vi "Thermal Shock.vi"() -> ()   [LabVIEW 2017]
uses:
  StateDef.ctl
  Thermal Shock.lvlib
panel:
  in  "Tab Control":enum32{"Main Program", "Graph", "Debug"}(tab)
  in  "ProgramTemp":bool
  in  "StopCycling":bool
  in  "StartCycling":bool
  in  "StartChamber":enum32{"Hot", "Cold"}(radio) caption="Starting Chamber"
  in  "Number of Cycles":u32
  in  "Basket Control":enum32{"Basket Up", "Basket Down"}(radio)=enum."Basket Down"
  in  "Stop Recording":bool
  in  "StartRecording":bool
  in  "Recording Interval":T1
  in  "Recording Duration":T2
  in  "Close Program":bool
  out "experiorLogo":picture
  out "Test Information":T3
  in  "HotSetPoint":i32 caption="Hot Chamber Temp (°C)"
  in  "ColdSetPoint":i32 caption="Cold Chamber Temp (°C)"
  in  "ChamberDwells":T4 {"sec_HotDwell" max=60}
  out "TempChart":cluster{"Value":dbl, "Value":i32}[](graph)
  out "Cold Chamber Set Command":string
  out "Hot Chamber Set Command":string
  out "Chamber Dwell Params":u32[](array[numeric])
  out "DataFilePath":path
  in  "Current Temperature":i32[](array[numeric])
  in  "Time (hours)":dbl[](array[numeric])
  out "ElapsedTimeHours":dbl
  out "CurrentColdTemp":i32
  out "CurrentHotTemp":i32
  out "UpdateGraph":bool
  out "FileCreated":bool
  out "CurrentCycle":u32
  out "CycleStartTime":u32
  out "StartTimeDuration":u32
  out "NumberCycles":u32
  out "ColdDwell":u32
  out "HotDwell":u32
  out "Cycling":bool
  out "Close Data Loop":bool
  out "Basket State":u32
  out "Temperature Readings":T5
  out "Data Recording":bool
  out "Recording Interval and Duration":u32[](array[numeric]) caption="MeasParams"
  out "Termination Message":string
  out "Simulated Data":bool
  in  "Queue Cluster":T7
  out "error out":errorcluster
  out "refnum out":refnum<file>
  out "StartTime":u32
  # "File Recording Setup"
  # "Temperature Control"
  # "Cycle Control"
  # "Basket Control"
  # "Data File Information"
  # "Hot Chamber Dwell"
  # "Cold Chamber Dwell"
  # "Temperature Graph"
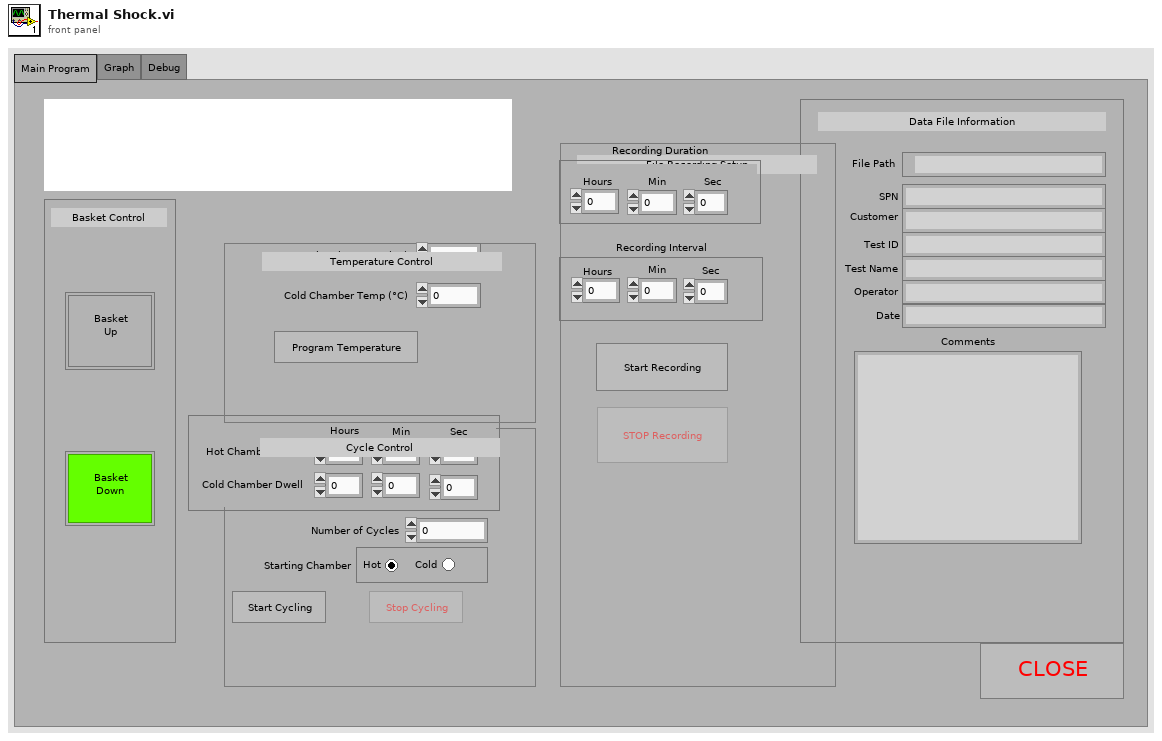
[diagram p1: front panel]
types:
  T1 = cluster{"hours_Interval":i16, "min_Duration":i16, "sec_Duration":i16}
  T2 = cluster{"hours_Duration":u16, "min_Duration":u16, "sec_Duration":i16}
  T3 = cluster{"Test ID":string, "Test Name":string, "Customer":string, "SPN":string, "Operator":string, "Date":string, "File Path":path, "Comments":string}
  T4 = cluster{"hours_HotDwell":u32, "min_HotDwell":u32, "sec_HotDwell":u32, "sec_ColdDwell":u32, "min_ColdDwell":u32, "hours_ColdDwell":u32}
  T5 = cluster{"HotChamber":string, "ColdChamber":string, "Time":string, "Date":string}
  T6 = typedef "StateDef.ctl" = enum16{"Timeout", "AppendFileHeaders", "StopRecording", "TestInformation", "Terminate", "Initialize", "StartRecording", "ReadInstruments", "ReadTemperature", "WriteData", "StartCycling", "StopCycling", "ProgramTemperatures", "CycleBasket"}
  T7 = cluster{"Enum":T6, "Error Note":string, "Message Data":variant}
  T8 = enum8{"Enabled", "Disabled", "Disabled and Grayed Out"}
  T9 = enum16{"open", "replace", "create", "open or create", "replace or create", "replace or create with confirmation"}
  T10 = cluster{string, string, string, string, string, string, path, string}
  T11 = cluster{"Enum":T6, string, "Message Data":variant}
  T12 = cluster{"Test ID":string, "Test Name":string, "Customer":string, "SPN":string, "Operator Name":string, "Date":string, "File Path":path, "Comments":string}
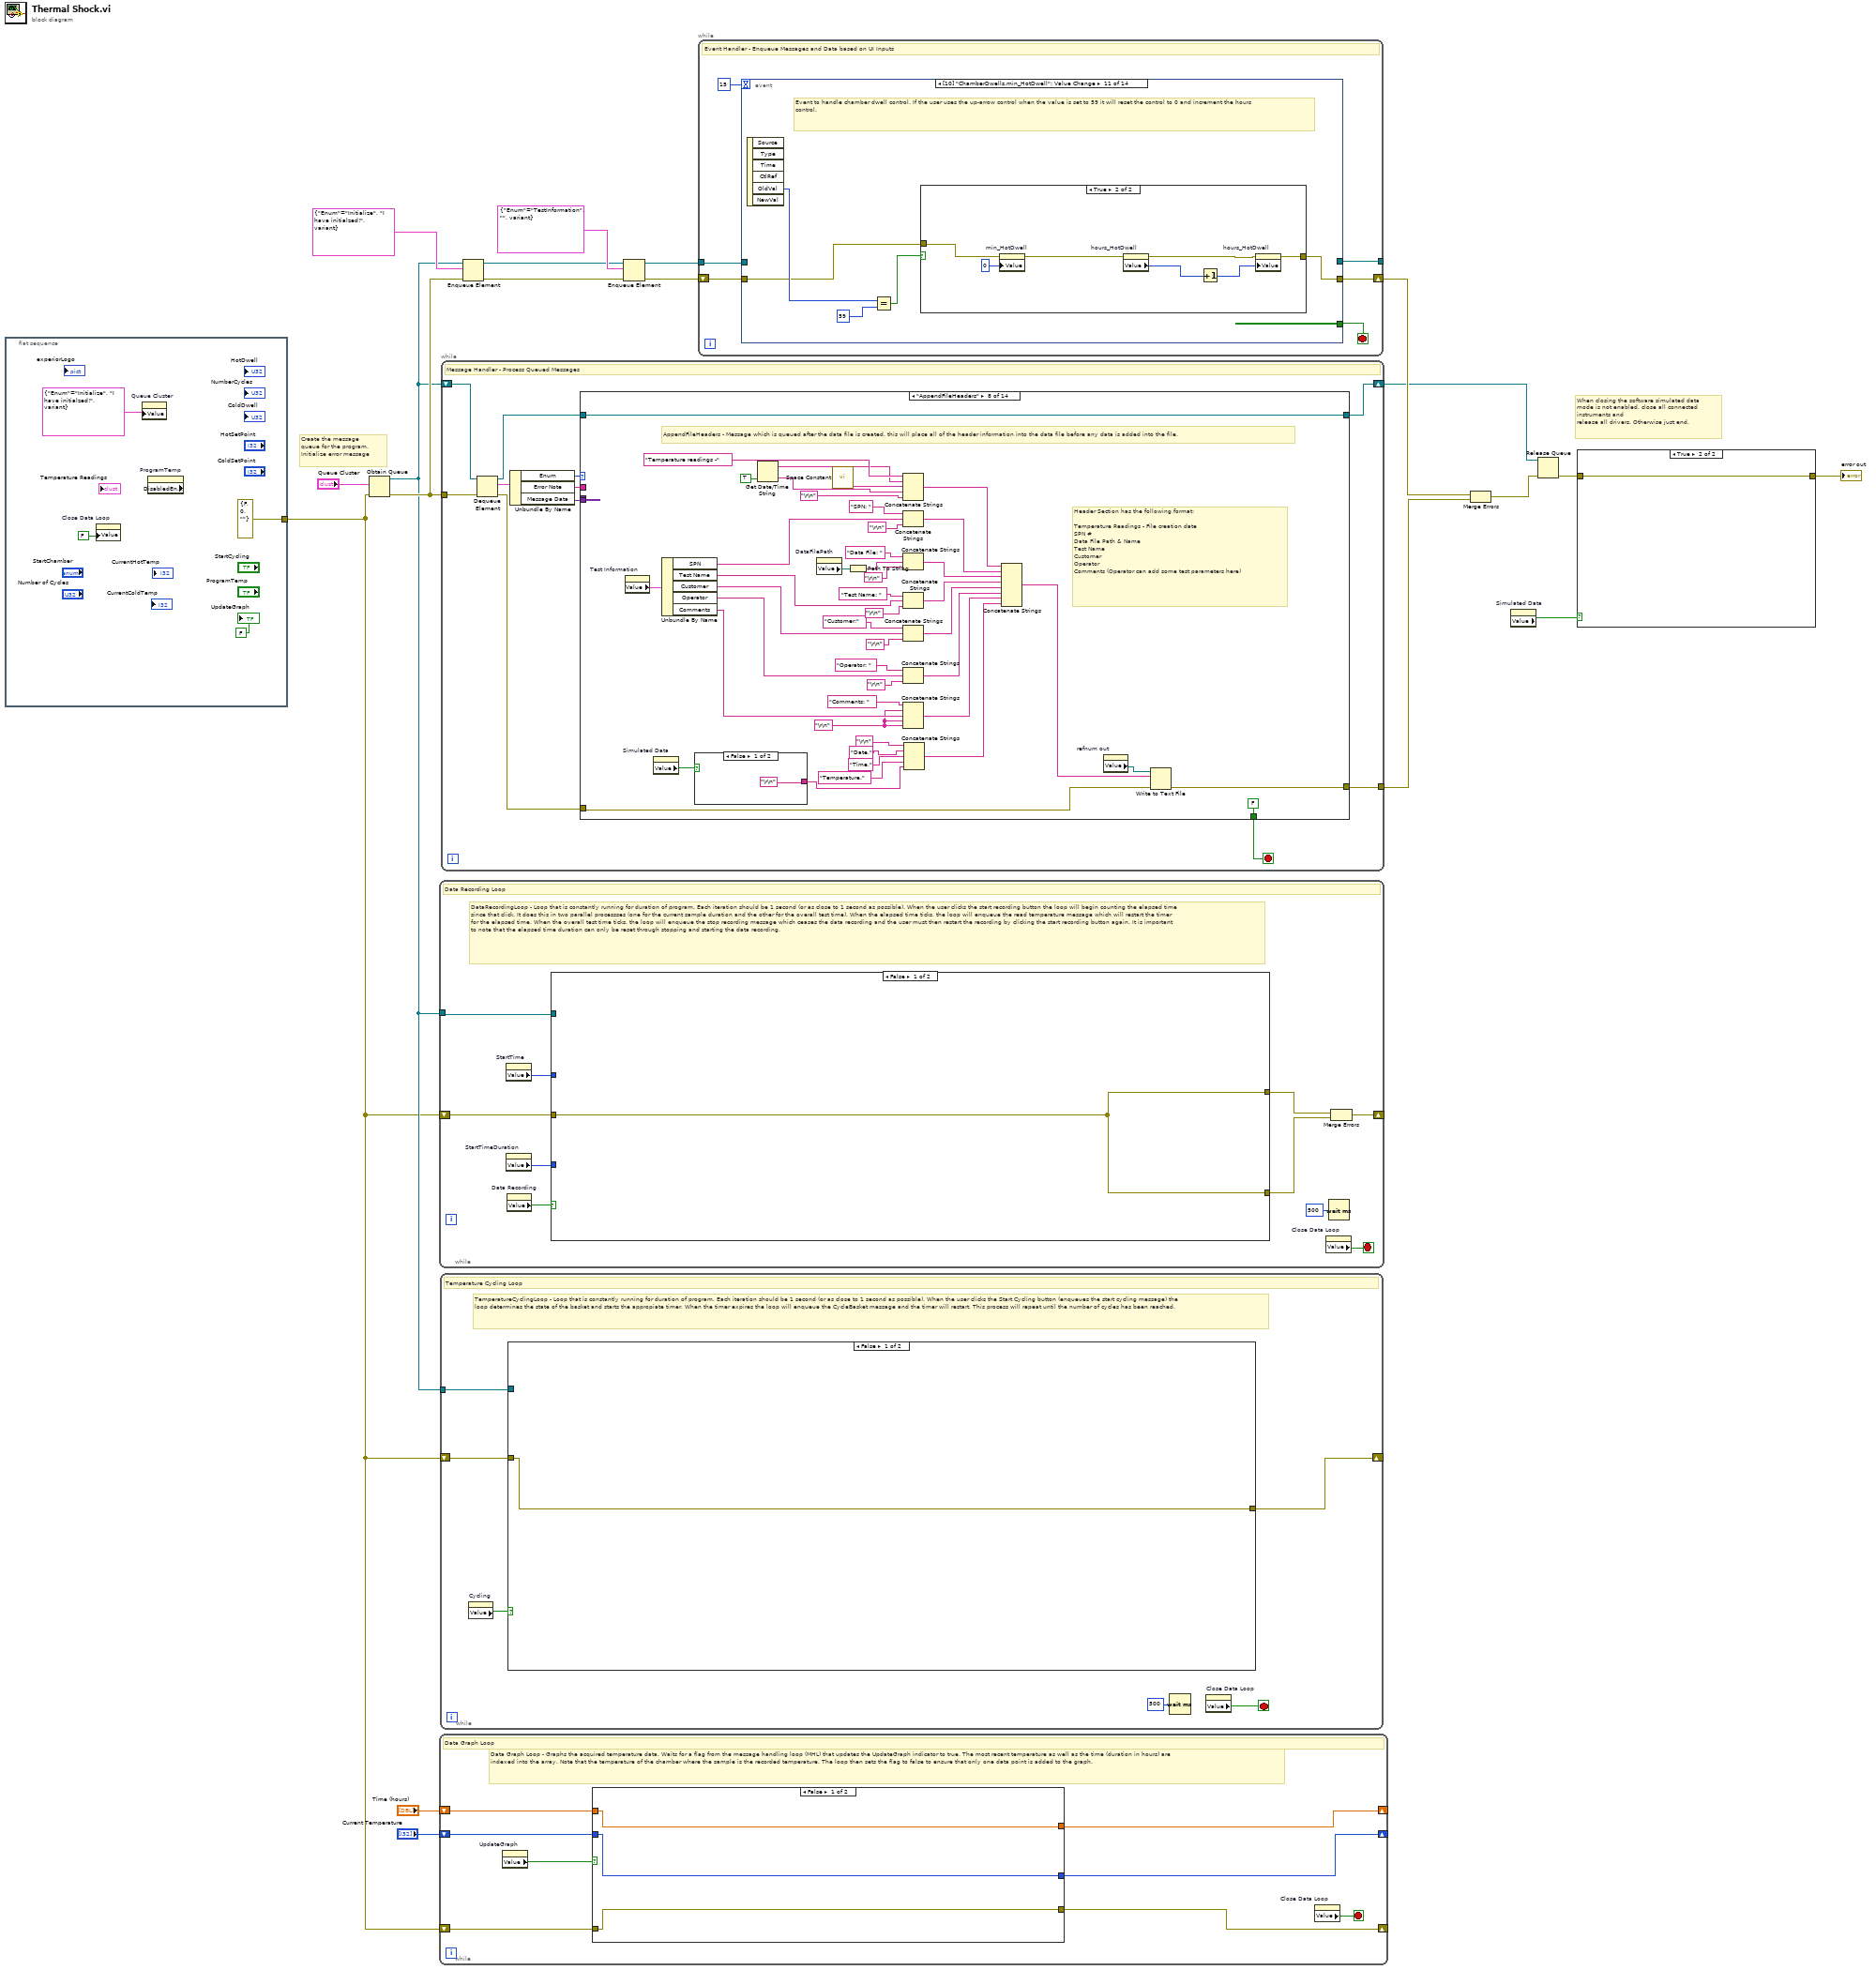
[diagram p0: block diagram]
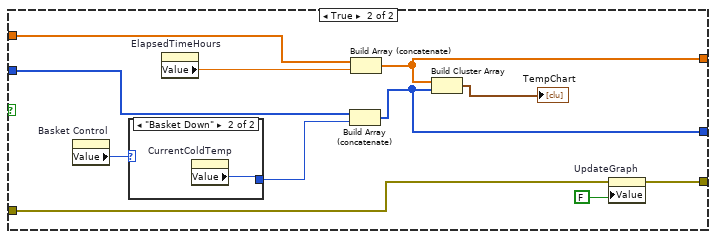
[diagram p2: hidden frame]
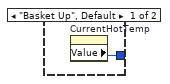
[diagram p3: hidden frame]
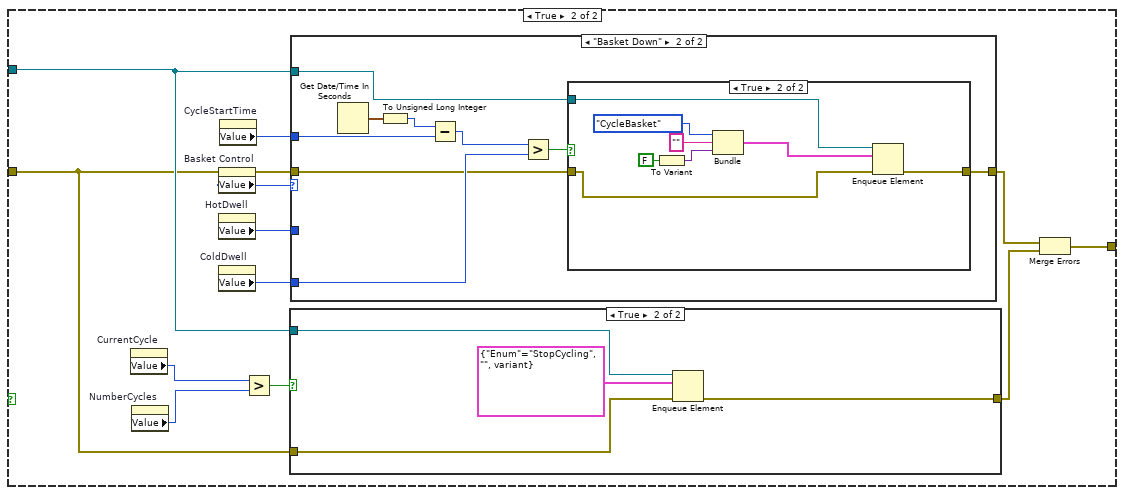
[diagram p4: hidden frame]
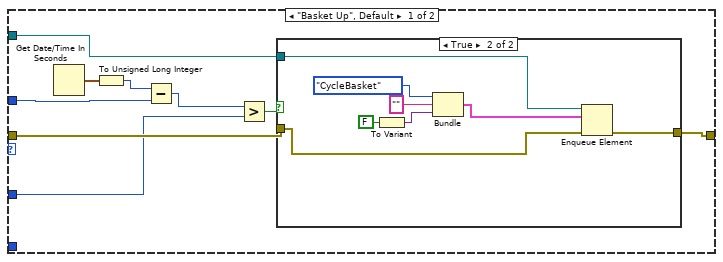
[diagram p6: hidden frame]
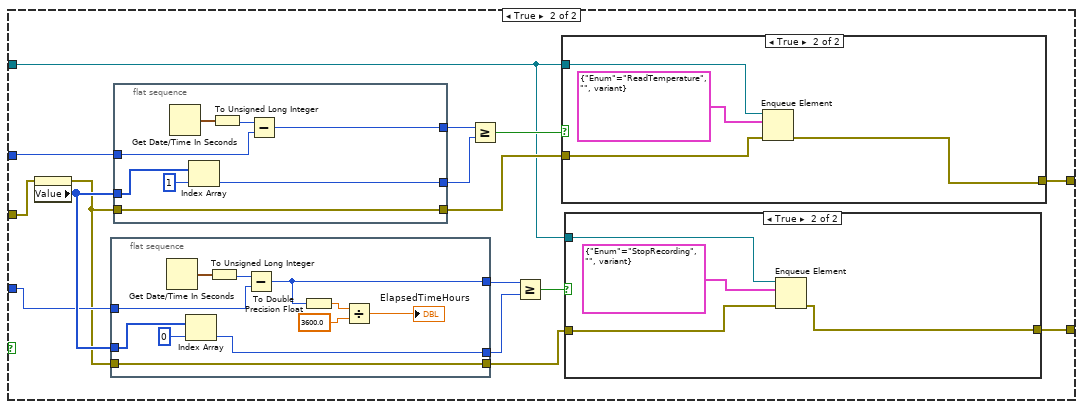
[diagram p9: hidden frame]
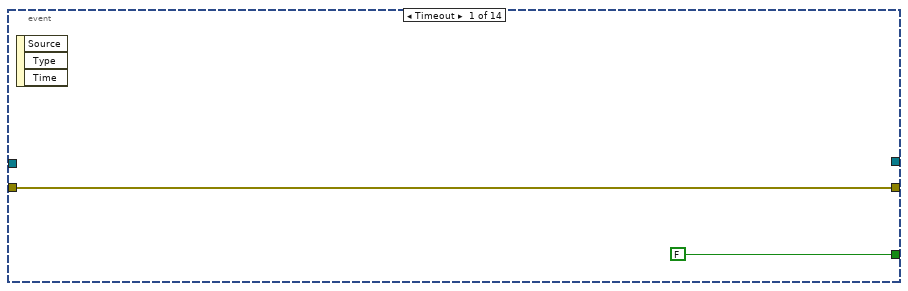
[diagram p13: hidden frame]
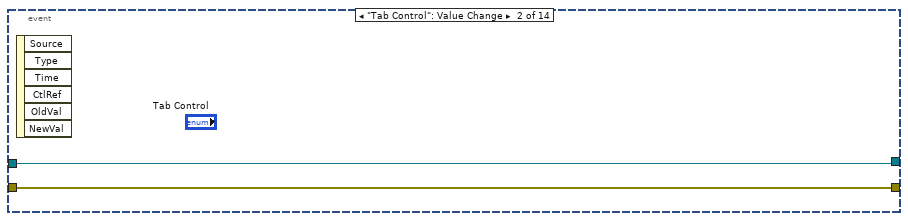
[diagram p14: hidden frame]
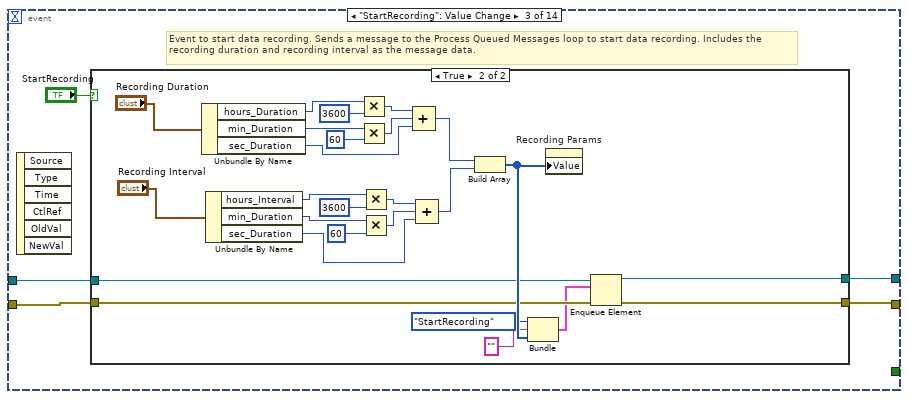
[diagram p15: hidden frame]
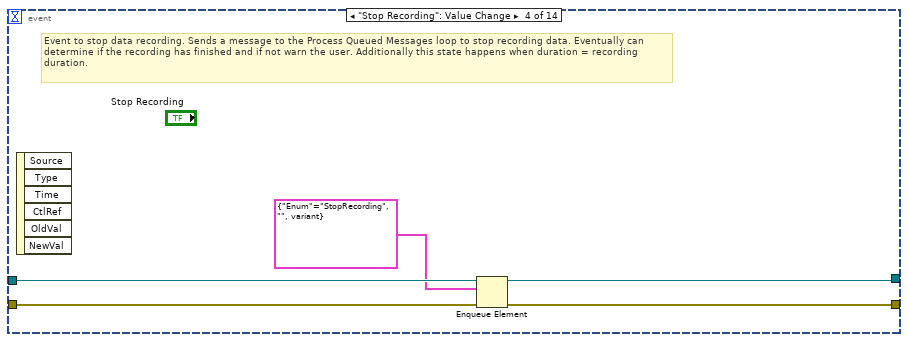
[diagram p17: hidden frame]
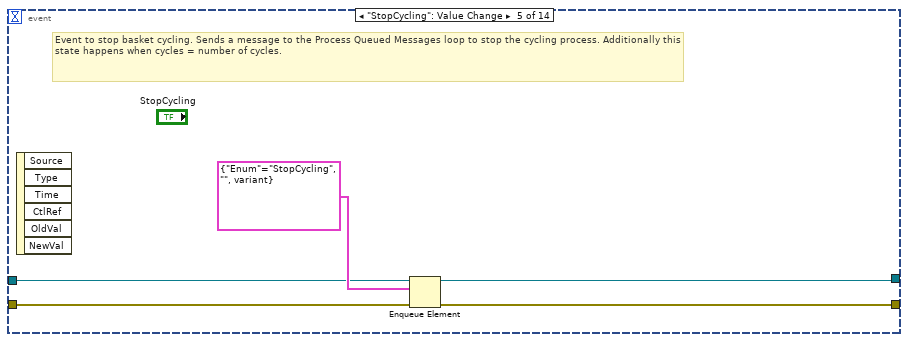
[diagram p18: hidden frame]
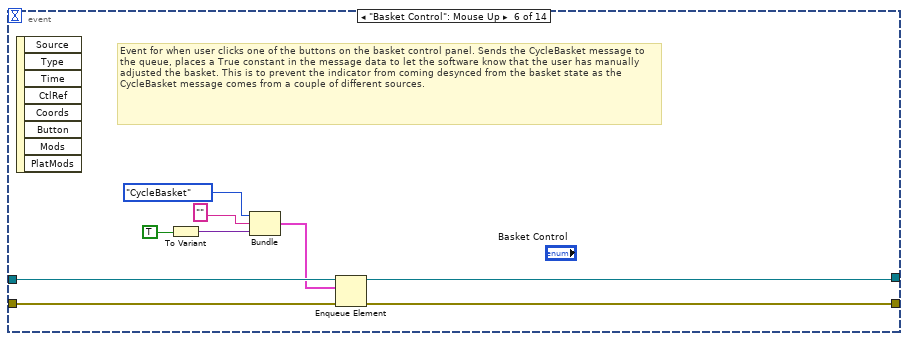
[diagram p19: hidden frame]
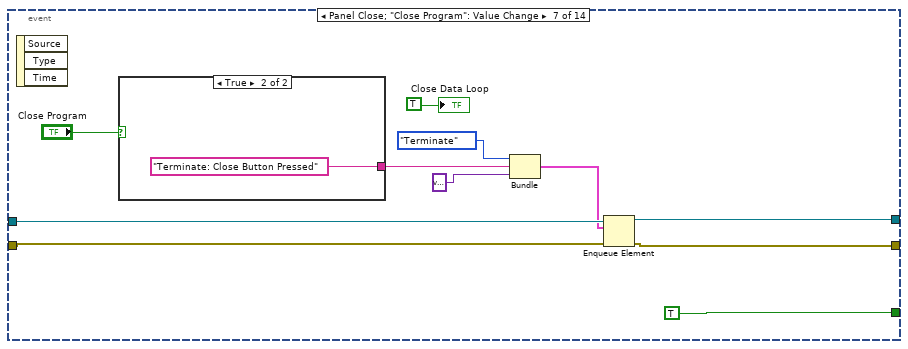
[diagram p20: hidden frame]
diagram:
  # "When closing the software simulated data mode is not enabled, close all connected instruments and \nrelease all drivers. Otherwise just end."
  # "Create the message queue for the program. Initialize error message"
  n1 = flat-sequence {
    tunnel: [errorcluster {"status"=FALSE, "code"=0, "source"=""} ("error constant")] -> w3
    frame #0 {
      n2 = property on="Close Data Loop" class="Bool (strict)"("Value"=FALSE) -> ()  [unwired: 2 in, 2 out]
      n3 = property on="Queue Cluster" class="Clust (strict)"("Value"=cluster{"Enum":T6, string, variant} {"Enum"=enum."Initialize", "I have initialzed!", variant}) -> ()  [unwired: 2 in, 2 out]
      n4 = property on="ProgramTemp" class="Bool" props=["DisabledEnum"]() -> ()  [unwired: 2 in, 3 out]
      "UpdateGraph" <- FALSE ("UpdateGraph")
    }
  }
  n5 = Obtain Queue(element data type="Queue Cluster", error in (no error)=w3) -> (queue out=w4:refnum<queue>, error out=w6:errorcluster)  [unwired: 3 in, 1 out]
  n6 = while {
    shift-right: [w24] -> _
    shift-left: w3 -> [w32]
    tunnel: w4 -> [w31]
    stop <- w28 stop-if-true
    # "DataRecordingLoop - Loop that is constantly running for duration of program. Each iteration should be 1 second (or as close to 1 second as possible). When the user clicks the start recording button the loop will begin counting the elapsed time since that click. It does this in two parallel processses (one for the current sample duration and the other for the overall test time). When the elapsed time ticks, the loop will enqueue the read temperature message which will restart the timer for the elapsed time. When the overall test time ticks, the loop will enqueue the stop recording message which ceases the data recording and the user must then restart the recording by clicking the start recording button again. It is important to note that the elapsed time duration can only be reset through stopping and starting the data recording."
    # "Data Recording Loop"
    n7 = property on="StartTime" class="DigNum (strict)"() -> ("Value"=w29:u32)  [unwired: 2 in, 2 out]
    n8 = property on="StartTimeDuration" class="DigNum (strict)"() -> ("Value"=w27:u32)  [unwired: 2 in, 2 out]
    n9 = property on="Data Recording" class="Bool (strict)"() -> ("Value"=w33:bool)  [unwired: 2 in, 2 out]
    n10 = case shown="False" w33 {
      tunnel: w29 -> [_ w48]
      tunnel: w32 -> [w34 w50]
      tunnel: w31 -> [_ w38]
      tunnel: [w34 w47] -> w26
      tunnel: w27 -> [_ w43]
      tunnel: [w34 w36] -> w25
      frame False {
      }
      frame True {
        n11 = property on="Recording Interval and Duration" class="Arr (strict)"(error in=w50) -> (error out=w42:errorcluster, "Value"=w44:u32[])  [unwired: 1 in, 1 out]
        n12 = flat-sequence {
          tunnel: [w59] -> w41
          tunnel: w43 -> [w64]
          tunnel: w42 -> [w60]
          tunnel: w44 -> [w62]
          tunnel: [w61] -> w40
          tunnel: [w60] -> w37
          frame #0 {
            n13 = Get Date/Time In Seconds() -> (seconds since 1Jan1904=w66:timestamp)
            n14 = Index Array(array=w62, index=0) -> (element=w61:u32)
            n15 = To Unsigned Long Integer(number=w66) -> (unsigned 32bit integer=w65:u32)
            n16 = Subtract(x=w65, y=w64) -> (x-y=w59:u32)
            n17 = To Double Precision Float(number=w59) -> (double precision float=w58:dbl)
            n18 = Divide(x=w58, y=3600.0) -> (x/y=→"ElapsedTimeHours":dbl)
          }
        }
        n19 = flat-sequence {
          tunnel: [w73] -> w35
          tunnel: w48 -> [w71]
          tunnel: w42 -> [w70]
          tunnel: [w70] -> w46
          tunnel: w44 -> [w68]
          tunnel: [w67] -> w45
          frame #0 {
            n20 = Get Date/Time In Seconds() -> (seconds since 1Jan1904=w74:timestamp)
            n21 = Index Array(array=w68, index=1) -> (element=w67:u32)
            n22 = To Unsigned Long Integer(number=w74) -> (unsigned 32bit integer=w72:u32)
            n23 = Subtract(x=w72, y=w71) -> (x-y=w73:u32)
          }
        }
        n24 = Greater Or Equal?(x=w35, y=w45) -> (x >= y?=w49:bool)
        n25 = Greater Or Equal?(x=w41, y=w40) -> (x >= y?=w39:bool)
        n26 = case shown="True" w49 {
          tunnel: w46 -> [w75 w78]
          tunnel: w38 -> [_ w79]
          tunnel: [w75 w77] -> w47
          frame False {
          }
          frame True {
            n27 = Enqueue Element(queue=w79, element=cluster{"Enum":T6, string, variant} {"Enum"=enum."ReadTemperature", "", variant}, error in (no error)=w78) -> (error out=w77:errorcluster)  [unwired: 1 in, 2 out]
          }
        }
        n28 = case shown="True" w39 {
          tunnel: w38 -> [_ w55]
          tunnel: w37 -> [w51 w53]
          tunnel: [w51 w52] -> w36
          frame False {
          }
          frame True {
            n29 = Enqueue Element(queue=w55, element=cluster{"Enum":T6, string, variant} {"Enum"=enum."StopRecording", "", variant}, error in (no error)=w53) -> (error out=w52:errorcluster)  [unwired: 1 in, 2 out]
          }
        }
      }
    }
    n30 = property on="Close Data Loop" class="Bool (strict)"() -> ("Value"=w28:bool)  [unwired: 2 in, 2 out]
    n31 = Wait (ms)(milliseconds to wait=u32 500) -> ()  [unwired: 1 out]
    n32 = Merge Errors(w26, w25) -> (w24:errorcluster)
  }
  n33 = while {
    shift-right: [w84] -> _
    shift-left: w3 -> [w85]
    shift-right: [w80] -> _
    shift-left: "Current Temperature" -> [w82]
    shift-right: [w81] -> _
    shift-left: "Time (hours)" -> [w83]
    stop <- w87 stop-if-true
    # "Data Graph Loop - Graphs the acquired temperature data. Waits for a flag from the message handling loop (MHL) that updates the UpdateGraph indicator to true. The most recent temperature as well as the time (duration in hours) are indexed into the array. Note that the temperature of the chamber where the sample is the recorded temperature. The loop then sets the flag to false to ensure that only one data point is added to the graph."
    # "Data Graph Loop"
    n34 = property on="UpdateGraph" class="Bool (strict)"() -> ("Value"=w86:bool)  [unwired: 2 in, 2 out]
    n35 = case shown="False" w86 {
      tunnel: w85 -> [w90 w100]
      tunnel: [w90 w99] -> w84
      tunnel: w83 -> [w88 w98]
      tunnel: w82 -> [w89 w96]
      tunnel: [w88 w94] -> w81
      tunnel: [w89 w93] -> w80
      frame False {
      }
      frame True {
        n36 = property on="Basket Control" class="RadioBtnsControl (strict)"() -> ("Value"=w91:enum32{"Basket Up", "Basket Down"})  [unwired: 2 in, 2 out]
        n37 = case shown="\"Basket Down\"" w91 {
          tunnel: [w102 w103] -> w95
          frame "Basket Up", Default {
            n38 = property on="CurrentHotTemp" class="DigNum (strict)"() -> ("Value"=w102:i32)  [unwired: 2 in, 2 out]
          }
          frame "Basket Down" {
            n39 = property on="CurrentColdTemp" class="DigNum (strict)"() -> ("Value"=w103:i32)  [unwired: 2 in, 2 out]
          }
        }
        n40 = property on="ElapsedTimeHours" class="DigNum (strict)"() -> ("Value"=w97:dbl)  [unwired: 2 in, 2 out]
        n41 = Build Array (concatenate)(w96, w95) -> (w93:i32[])
        n42 = Build Array (concatenate)(w98, w97) -> (w94:dbl[])
        n43 = Build Cluster Array(w94, w93) -> (→"TempChart":cluster{"Value":dbl, "Value":i32}[])
        n44 = property on="UpdateGraph" class="Bool (strict)"(error in=w100, "Value"=FALSE) -> (error out=w99:errorcluster)  [unwired: 1 in, 1 out]
      }
    }
    n45 = property on="Close Data Loop" class="Bool (strict)"() -> ("Value"=w87:bool)  [unwired: 2 in, 2 out]
  }
  n46 = while {
    tunnel: w4 -> [w107]
    shift-right: [w104] -> _
    shift-left: w3 -> [w106]
    stop <- w109 stop-if-true
    # "TemperatureCyclingLoop - Loop that is constantly running for duration of program. Each iteration should be 1 second (or as close to 1 second as possible). When the user clicks the Start Cycling button (enqueues the start cycling message) the loop determines the state of the basket and starts the appropiate timer. When the timer expires the loop will enqueue the CycleBasket message and the timer will restart. This process will repeat until the number of cycles has been reached."
    # "Temperature Cycling Loop"
    n47 = property on="Cycling" class="Bool (strict)"() -> ("Value"=w105:bool)  [unwired: 2 in, 2 out]
    n48 = case shown="False" w105 {
      tunnel: w107 -> [_ w115]
      tunnel: w106 -> [w110 w114]
      tunnel: [w110 w111] -> w104
      frame False {
      }
      frame True {
        n49 = property on="CurrentCycle" class="DigNum (strict)"() -> ("Value"=w118:u32)  [unwired: 2 in, 2 out]
        n50 = property on="NumberCycles" class="DigNum (strict)"() -> ("Value"=w117:u32)  [unwired: 2 in, 2 out]
        n51 = property on="Basket Control" class="RadioBtnsControl (strict)"(error in=w114) -> (error out=w119:errorcluster, "Value"=w123:enum32{"Basket Up", "Basket Down"})  [unwired: 1 in, 1 out]
        n52 = property on="HotDwell" class="DigNum (strict)"() -> ("Value"=w121:u32)  [unwired: 2 in, 2 out]
        n53 = property on="ColdDwell" class="DigNum (strict)"() -> ("Value"=w120:u32)  [unwired: 2 in, 2 out]
        n54 = property on="CycleStartTime" class="DigNum (strict)"() -> ("Value"=w122:u32)  [unwired: 2 in, 2 out]
        n55 = Greater?(x=w118, y=w117) -> (0:w116:bool)
        n56 = case shown="True" w116 {
          tunnel: w115 -> [_ w127]
          tunnel: w114 -> [w124 w126]
          tunnel: [w124 w125] -> w112
          frame False {
          }
          frame True {
            n57 = Enqueue Element(queue=w127, element=cluster{"Enum":T6, string, variant} {"Enum"=enum."StopCycling", "", variant}, error in (no error)=w126) -> (error out=w125:errorcluster)  [unwired: 1 in, 2 out]
          }
        }
        n58 = case shown="\"Basket Down\"" w123 {
          tunnel: w122 -> [w129 w153]
          tunnel: w121 -> [w131 _]
          tunnel: w120 -> [_ w151]
          tunnel: w115 -> [w133 w149]
          tunnel: w119 -> [w132 w148]
          tunnel: [w130 w147] -> w113
          frame "Basket Up", Default {
            n59 = Get Date/Time In Seconds() -> (seconds since 1Jan1904=w137:timestamp)
            n60 = To Unsigned Long Integer(number=w137) -> (unsigned 32bit integer=w136:u32)
            n61 = Subtract(x=w136, y=w129) -> (x-y=w135:u32)
            n62 = Greater?(x=w135, y=w131) -> (0:w134:bool)
            n63 = case shown="True" w134 {
              tunnel: w133 -> [_ w145]
              tunnel: w132 -> [w138 w146]
              tunnel: [w138 w144] -> w130
              frame False {
              }
              frame True {
                n64 = To Variant(anything=FALSE) -> (Variant=w141:variant)
                n65 = Bundle("Enum"=StateDef."CycleBasket", "", "Variant"=w141) -> (w139:cluster{"Enum":T6, string, "Variant":variant})  [unwired: 1 in]
                n66 = Enqueue Element(queue=w145, element=w139, error in (no error)=w146) -> (error out=w144:errorcluster)  [unwired: 1 in, 2 out]
              }
            }
          }
          frame "Basket Down" {
            n67 = Get Date/Time In Seconds() -> (seconds since 1Jan1904=w155:timestamp)
            n68 = To Unsigned Long Integer(number=w155) -> (unsigned 32bit integer=w154:u32)
            n69 = Subtract(x=w154, y=w153) -> (x-y=w152:u32)
            n70 = Greater?(x=w152, y=w151) -> (0:w150:bool)
            n71 = case shown="True" w150 {
              tunnel: w149 -> [_ w163]
              tunnel: w148 -> [w156 w164]
              tunnel: [w156 w162] -> w147
              frame False {
              }
              frame True {
                n72 = To Variant(anything=FALSE) -> (Variant=w158:variant)
                n73 = Bundle("Enum"=StateDef."CycleBasket", "", "Variant"=w158) -> (w157:cluster{"Enum":T6, string, "Variant":variant})  [unwired: 1 in]
                n74 = Enqueue Element(queue=w163, element=w157, error in (no error)=w164) -> (error out=w162:errorcluster)  [unwired: 1 in, 2 out]
              }
            }
          }
        }
        n75 = Merge Errors(w113, w112) -> (w111:errorcluster)
      }
    }
    n76 = Wait (ms)(milliseconds to wait=u32 500) -> ()  [unwired: 1 out]
    n77 = property on="Close Data Loop" class="Bool (strict)"() -> ("Value"=w109:bool)  [unwired: 2 in, 2 out]
  }
  n78 = while {
    shift-right: [w166] -> w13
    shift-left: w4 -> [w175]
    tunnel: w6 -> [w170]
    tunnel: [w168] -> w14
    stop <- w171 stop-if-true
    # "Message Handler - Process Queued Messages"
    n79 = Dequeue Element(queue=w175, error in (no error)=w170) -> (queue out=w167:refnum<queue>, element=w174:T7, error out=w169:errorcluster)  [unwired: 1 in, 1 out]
    n80 = Unbundle By Name(w174) -> ("Enum"=w173:T6, "Error Note"=w172:string, "Message Data"=w165:variant)
    n81 = case shown="\"AppendFileHeaders\"" w173 {
      tunnel: w172 -> [_ w184 _ _ _ _ _ _ _ _ _ _ _ _]
      tunnel: w165 -> [_ _ _ w226 w257 w327 _ _ w462 w485 _ _ _ _]
      tunnel: [FALSE TRUE FALSE FALSE FALSE FALSE FALSE FALSE FALSE FALSE FALSE FALSE FALSE FALSE] -> w171
      tunnel: w169 -> [w177 w182 w209 w225 w263 w325 w360 w407 w464 w479 w524 w531 w551 w558]
      tunnel: [w177 w179 w209 w231 w256 w301 w340 w439 w453 w476 w524 w525 w549 w555] -> w168
      tunnel: w167 -> [w176 w183 w210 w232 w259 w304 w357 w440 w459 w488 w522 w533 w546 w554]
      tunnel: [w176 w183 w210 w232 w255 w304 w339 w440 w459 w488 w522 w533 w546 w554] -> w166
      tunnel: w165 -> [_ _ _ _ _ _ _ _ _ _ _ _ _ _]
      frame "Timeout", Default {
      }
      frame "Terminate" {
        # "Terminate - Message when the program is closed. Closes any open data files and shuts down all running loops (EHL, MHL, DRL, TCL, DGL). Can add other shutdown procedures here later."
        n82 = property on="FileCreated" class="Bool (strict)"(error in=w182) -> (error out=w180:errorcluster, "Value"=w181:bool)  [unwired: 1 in, 1 out]
        n83 = case shown="True" w181 {
          tunnel: w180 -> [w186 w190]
          tunnel: [w186 w188] -> w179
          frame False {
          }
          frame True {
            n84 = property on="refnum out" class="Ref (strict)"() -> ("Value"=w191:refnum<file>)  [unwired: 2 in, 2 out]
            n85 = Close File(refnum=w191, error in=w190) -> (error out=w189:errorcluster)  [unwired: 1 out]
            n86 = property on="FileCreated" class="Bool (strict)"(error in=w189, "Value"=FALSE ("FileCreated")) -> (error out=w188:errorcluster)  [unwired: 1 in, 1 out]
          }
        }
        n87 = property on="Termination Message" class="Str"("Value"=w184) -> ()  [unwired: 2 in, 2 out]
      }
      frame "Initialize" {
        w211 = FALSE ("Simulated Data")
        w215 = ""
        w219 = u32 1
        w207 = u32 0
        # "Initialize Message - This is the first message processed after starting the program. Applies initial conditions for all relevant controls and indicators. Controls are grouped together in the various blocks."
        n88 = property on="Close Program" class="Bool (strict)"("Value"=FALSE) -> ()  [unwired: 2 in, 2 out]
        n89 = Bundle(w219, w207, w207) -> (w218:cluster{u32, u32, u32})  [unwired: 1 in]
        n90 = Bundle(w207, w219, w207) -> (w217:cluster{u32, u32, u32})  [unwired: 1 in]
        n91 = Bundle(u32 1, u32 30, u32 0, u32 0, u32 30, u32 0) -> (w198:cluster{u32, u32, u32, u32, u32, u32})  [unwired: 1 in]
        n92 = property on="Recording Duration" class="Clust (strict)"("Value"=w218) -> ()  [unwired: 2 in, 2 out]
        n93 = property on="Recording Interval" class="Clust (strict)"("Value"=w217) -> ()  [unwired: 2 in, 2 out]
        n94 = property on="Simulated Data" class="Bool (strict)"("Value"=w211) -> ()  [unwired: 2 in, 2 out]
        n95 = property on="ChamberDwells" class="Clust (strict)"("Value"=w198) -> ()  [unwired: 2 in, 2 out]
        n96 = property on="Number of Cycles" class="DigNum (strict)"("Value"=u32 10 ("Number of Cycles")) -> ()  [unwired: 2 in, 2 out]
        n97 = property on="StartChamber" class="RadioBtnsControl (strict)"("Value"=enum32{"Hot", "Cold"}."Hot" ("StartChamber")) -> ()  [unwired: 2 in, 2 out]
        n98 = Bundle(w215, w215, w215, w215, w215, w215, path "", w215) -> (w214:T10)  [unwired: 1 in]
        n99 = property on="StartRecording" class="Bool"("DisabledEnum"=T8."Enabled" ("Disabled")) -> ()  [unwired: 2 in, 2 out]
        n100 = property on="Stop Recording" class="Bool (strict)"("DisabledEnum"=T8."Disabled and Grayed Out" ("Disabled")) -> ()  [unwired: 2 in, 2 out]
        n101 = property on="Test Information" class="Clust (strict)"("Value"=w214) -> ()  [unwired: 2 in, 2 out]
        n102 = property on="StopCycling" class="Bool (strict)"("DisabledEnum"=T8."Disabled and Grayed Out" ("Disabled")) -> ()  [unwired: 2 in, 2 out]
        n103 = property on="StartCycling" class="Bool (strict)"("DisabledEnum"=T8."Enabled" ("Disabled")) -> ()  [unwired: 2 in, 2 out]
        n104 = property on="ColdSetPoint" class="DigNum (strict)"("Value"=10 ("ColdSetPoint")) -> ()  [unwired: 2 in, 2 out]
        n105 = property on="HotSetPoint" class="DigNum (strict)"("Value"=35 ("HotSetPoint")) -> ()  [unwired: 2 in, 2 out]
        "Termination Message" <- ""
        "Data Recording" <- w211
        "Cycling" <- FALSE
        "FileCreated" <- FALSE
      }
      frame "ProgramTemperatures" {
        w227 = 0
        # "ProgramTemperatures - Message which attempts to send the values in the Temperature Control block to the Chromalox controller. The message data is in the format of a 2 Integer cluster with the following structure:\n\nI32[0] = Hot Chamber Temperature\nI32[1] = Cold Chamber Temperature\n\nNote that when the Simulated Data control is enabled this message does nothing (no good way to enable debugging for this method)."
        n106 = property on="Simulated Data" class="Bool (strict)"() -> ("Value"=w233:bool)  [unwired: 2 in, 2 out]
        n107 = Bundle(w227, w227) -> (w228:cluster{i32, i32})  [unwired: 1 in]
        n108 = Variant To Data(error in=w225, type=w228, Variant=w226) -> (data=w229:cluster{i32, i32}, error out=w224:errorcluster)
        n109 = Unbundle(w229) -> (w223:i32, w222:i32)
        n110 = case shown="True" w233 {
          tunnel: w224 -> [w234 w249]
          tunnel: [w237 w249] -> w231
          tunnel: w223 -> [w236 w248]
          tunnel: w222 -> [w235 w247]
          frame False {
            n111 = call "SetHighPoint.vi"("error in (no error)"=w234, "High Temperature"=w236) -> ("error out"=w238:errorcluster)  [unwired: 8 in, 1 out]
            n112 = call "SetLowPoint.vi"("error in (no error)"=w238, "Low Temperature"=w235) -> ("error out"=w237:errorcluster)  [unwired: 8 in, 1 out]
          }
          frame True {
            n113 = call "FormatHexValue.vi"("Value"=w248) -> ("FormattedValue"=w246:string)  [unwired: 10 in]
            n114 = call "FormatHexValue.vi"("Value"=w247) -> ("FormattedValue"=w243:string)  [unwired: 10 in]
            n115 = Concatenate Strings("0108000101", w246) -> (w242:string)
            n116 = Concatenate Strings("0108000201", w243) -> (w241:string)
            n117 = call "ComputeChecksum.vi"("Input Command"=w242) -> ("Command Message"=→"Hot Chamber Set Command":string)  [unwired: 9 in, 1 out]
            n118 = call "ComputeChecksum.vi"("Input Command"=w241) -> ("Command Message"=→"Cold Chamber Set Command":string)  [unwired: 9 in, 1 out]
          }
        }
      }
      frame "StartCycling" {
        # "StartCycling Message - When this message is received the software checks that the basket is in the proper starting chamber, if it is not then it will queue the cycle basket message follwed by the start cycling message so that the basket will be put in the right position. Otherwise this message will start the cycling timer.  This message will also update the status boxes for the two different dwell times and the number of cycles to keep track of where the program is."
        n119 = property on="Basket Control" class="RadioBtnsControl (strict)"() -> ("Value"=w254:enum32{"Basket Up", "Basket Down"})  [unwired: 2 in, 2 out]
        n120 = property on="StartChamber" class="RadioBtnsControl (strict)"() -> ("Value"=w253:enum32{"Hot", "Cold"})  [unwired: 2 in, 2 out]
        n121 = property on="StartCycling" class="Bool (strict)"(error in=w263, "DisabledEnum"=T8."Disabled and Grayed Out" ("Disabled")) -> (error out=w262:errorcluster)  [unwired: 1 in, 1 out]
        n122 = To Unsigned Long Integer(number=w254) -> (unsigned 32bit integer=w252:u32)
        n123 = To Unsigned Long Integer(number=w253) -> (unsigned 32bit integer=w251:u32)
        n124 = Equal?(x=w252, y=w251) -> (x = y?=w250:bool)
        n125 = property on="StopCycling" class="Bool (strict)"(error in=w262, "DisabledEnum"=T8."Enabled" ("Disabled")) -> (error out=w258:errorcluster)  [unwired: 1 in, 1 out]
        n126 = case shown="True" w250 {
          tunnel: w259 -> [w279 w290]
          tunnel: w258 -> [w278 w293]
          tunnel: [w271 w288] -> w256
          tunnel: w257 -> [w275 w291]
          tunnel: [w270 w290] -> w255
          frame False {
            n127 = To Variant(anything=FALSE) -> (Variant=w266:variant)
            n128 = Bundle("Enum"=StateDef."CycleBasket", "", "Variant"=w266) -> (w265:cluster{"Enum":T6, string, "Variant":variant})  [unwired: 1 in]
            n129 = Enqueue Element(queue=w279, element=w265, error in (no error)=w278) -> (queue out=w273:refnum<queue>, error out=w272:errorcluster)  [unwired: 1 in, 1 out]
            n130 = Bundle("Enum"=StateDef."StartCycling", "", "Message Data"=w275) -> (w274:T11)  [unwired: 1 in]
            n131 = Enqueue Element(queue=w273, element=w274, error in (no error)=w272) -> (queue out=w270:refnum<queue>, error out=w271:errorcluster)  [unwired: 1 in, 1 out]
          }
          frame True {
            n132 = property on="Chamber Dwell Params" class="Arr (strict)"() -> ("Value"=w287:u32[])  [unwired: 2 in, 2 out]
            n133 = Variant To Data(error in=w293, type=w287, Variant=w291) -> (data=w286:u32[], error out=w292:errorcluster)
            "Chamber Dwell Params" <- w286
            n134 = Index Array(array=w286, index #1=0 ("index"), index #2=1 ("index"), index #3=2 ("index")) -> (element #1=w282:u32, element #2=w281:u32, element #3=w280:u32)
            n135 = property on="Cycling" class="Bool (strict)"(error in=w292, "Value"=TRUE) -> (error out=w289:errorcluster)  [unwired: 1 in, 1 out]
            n136 = flat-sequence {
              tunnel: w289 -> [w296]
              tunnel: [w296] -> w288
              frame #0 {
                n137 = Get Date/Time In Seconds() -> (seconds since 1Jan1904=w297:timestamp)
                n138 = To Unsigned Long Integer(number=w297) -> (unsigned 32bit integer=→"CycleStartTime":u32)
                "CurrentCycle" <- u32 1
              }
            }
            n139 = property on="ColdDwell" class="DigNum (strict)"("Value"=w281) -> ()  [unwired: 2 in, 2 out]
            n140 = property on="HotDwell" class="DigNum (strict)"("Value"=w282) -> ()  [unwired: 2 in, 2 out]
            n141 = property on="NumberCycles" class="DigNum (strict)"("Value"=w280) -> ()  [unwired: 2 in, 2 out]
          }
        }
      }
      frame "StartRecording" {
        # "Take a timestamp for the start time. The data recording loop iterates every 500ms to check for a tick."
        # "Start Recording message, receives the recording (sampling) interval and recording (sampling) duration, both in seconds. Creates a new data file (csv) every time the start recording button is pressed, the file uses the time stamp to ensure a new file is created for each run. Sets the Data Recording indicator to true which will signal the data recording loop to begin processing."
        n142 = property on="Recording Interval and Duration" class="Arr (strict)"() -> ("Value"=w326:u32[])  [unwired: 2 in, 2 out]
        n143 = Variant To Data(error in=w325, type=w326, Variant=w327) -> (data=→"Recording Interval and Duration":u32[], error out=w313:errorcluster)
        n144 = property on="Test Information" class="Clust (strict)"() -> ("Value"=w322:T3)  [unwired: 2 in, 2 out]
        n145 = property on="StartRecording" class="Bool"(error in=w313, "DisabledEnum"=T8."Disabled and Grayed Out" ("Disabled")) -> (error out=w312:errorcluster)  [unwired: 1 in, 1 out]
        n146 = Unbundle By Name(w322) -> ("File Path"=w321:path, "SPN"=w316:string, "Test ID"=w309:string, "Test Name"=w308:string)
        n147 = call <vilib>:"Space Constant.vi"() -> ("String"=w307:string)
        n148 = Format Date/Time String(time format string (%c)="%Y%m%d%I%M%S") -> (date/time string=w306:string)  [unwired: 2 in]
        n149 = Path To String(path=w321) -> (string=w320:string)
        n150 = property on="Stop Recording" class="Bool (strict)"(error in=w312, "DisabledEnum"=T8."Enabled" ("Disabled")) -> (error out=w311:errorcluster)  [unwired: 1 in, 1 out]
        n151 = Concatenate Strings(w320, "\\", "SPN", w316, w307, w309, w307, w308, w307, w306, ".csv") -> (w318:string)
        n152 = String To Path(string=w318) -> (path=w299:path)
        "DataFilePath" <- w299
        n153 = Open/Create/Replace File(file path (use dialog)=w299, error in=w311, operation (0:open)=T9."create") -> (refnum out=→"refnum out":refnum<file>, error out=w303:errorcluster)  [unwired: 3 in, 1 out]
        n154 = Enqueue Element(queue=w304, element=cluster{"Enum":T6, string, variant} {"Enum"=enum."AppendFileHeaders", "", variant}, error in (no error)=w303) -> (error out=w302:errorcluster)  [unwired: 1 in, 2 out]
        n155 = flat-sequence {
          tunnel: w302 -> [w332]
          tunnel: [w332] -> w301
          frame #0 {
            n156 = Get Date/Time In Seconds() -> (seconds since 1Jan1904=w336:timestamp)
            n157 = Get Date/Time In Seconds() -> (seconds since 1Jan1904=w334:timestamp)
            n158 = To Unsigned Long Integer(number=w336) -> (unsigned 32bit integer=→"StartTime":u32)
            n159 = To Unsigned Long Integer(number=w334) -> (unsigned 32bit integer=→"StartTimeDuration":u32)
            n160 = property on="Data Recording" class="Bool (strict)"("Value"=TRUE) -> ()  [unwired: 2 in, 2 out]
            n161 = property on="FileCreated" class="Bool (strict)"("Value"=TRUE ("FileCreated")) -> ()  [unwired: 2 in, 2 out]
          }
        }
      }
      frame "ReadTemperature" {
        # "NOTE: The read commands for the Chromalox controller only return the offset from the set point temperature. This message reads the set point for each chamber and calculates the current temperature based on the offset. Can optimize by replacing the ReadHighSets with an indicator on the Main VI. \nNOTE2: Currently it seems like the Chromalox can only return/set integer values to/from the chamber. Legacy code was coded in a method that accounts for doubles however I could not find any data to support that. Looking into if this is a limitation of the controller or if there is a method for using doubles. Code is setup for calculating doubles however the values are just casted to 32 bit integers."
        # "Read Temperature Method - currently only called from a tick of the Data Recording Loop. Reads the temperature in the top and bottom chambers and creates a message from the two points. Enqueues the write data message to write the temperature to the data file. Built for expandability for collecting other types of data points."
        n162 = property on="Simulated Data" class="Bool (strict)"(error in=w360) -> (error out=w358:errorcluster, "Value"=w359:bool)  [unwired: 1 in, 1 out]
        n163 = case shown="False" w359 {
          tunnel: w358 -> [w367 w379]
          tunnel: w357 -> [w378 w380]
          tunnel: [w368 w382] -> w344
          tunnel: [w369 w381] -> w345
          tunnel: [w378 w380] -> w342
          tunnel: [w362 w379] -> w341
          frame False {
            n164 = call "ReadLowSetpoint.vi"("error in (no error)"=w367) -> ("error out"=w365:errorcluster, "LowChamberSetPoint"=w375:dbl)  [unwired: 7 in, 2 out]
            n165 = call "ReadHighSetpoint.vi"("error in (no error)"=w367) -> ("error out"=w366:errorcluster, "HighChamberSetPoint"=w377:dbl)  [unwired: 7 in, 2 out]
            n166 = call "ReadLowTemp.vi"("error in (no error)"=w365) -> ("error out"=w363:errorcluster, "CurrentTemp(LowChamber)"=w374:dbl)  [unwired: 7 in, 1 out]
            n167 = call "ReadHighTemp.vi"("error in (no error)"=w366) -> ("error out"=w364:errorcluster, "CurrentTemp(HighChamber)"=w376:dbl)  [unwired: 8 in, 1 out]
            n168 = Subtract(x=w377, y=w376) -> (x-y=w373:dbl)
            n169 = Subtract(x=w375, y=w374) -> (x-y=w372:dbl)
            n170 = To Long Integer(number=w373) -> (32bit integer=w371:i32)
            n171 = To Long Integer(number=w372) -> (32bit integer=w370:i32)
            n172 = Number To Decimal String(number=w371) -> (decimal integer string=w368:string)  [unwired: 1 in]
            n173 = Number To Decimal String(number=w370) -> (decimal integer string=w369:string)  [unwired: 1 in]
            n174 = Merge Errors(w364, w363) -> (w362:errorcluster)
          }
          frame True {
            n175 = Random Number (0-1)() -> (number: 0 to 1=w394:dbl)
            n176 = Random Number (0-1)() -> (number: 0 to 1=w393:dbl)
            n177 = property on="HotSetPoint" class="DigNum (strict)"() -> ("Value"=w388:i32)  [unwired: 2 in, 2 out]
            n178 = property on="ColdSetPoint" class="DigNum (strict)"() -> ("Value"=w386:i32)  [unwired: 2 in, 2 out]
            n179 = Multiply(x=w394, y=2.0) -> (x*y=w390:dbl)
            n180 = Multiply(x=w393, y=2.0) -> (x*y=w389:dbl)
            n181 = To Long Integer(number=w389) -> (32bit integer=w385:i32)
            n182 = To Long Integer(number=w390) -> (32bit integer=w387:i32)
            n183 = Add(x=w388, y=w387) -> (x+y=w384:i32)
            n184 = Add(x=w386, y=w385) -> (x+y=w383:i32)
            n185 = Number To Decimal String(number=w384) -> (decimal integer string=w382:string)  [unwired: 1 in]
            n186 = Number To Decimal String(number=w383) -> (decimal integer string=w381:string)  [unwired: 1 in]
            n187 = property on="CurrentColdTemp" class="DigNum (strict)"("Value"=w383) -> ()  [unwired: 2 in, 2 out]
            n188 = property on="CurrentHotTemp" class="DigNum (strict)"("Value"=w384) -> ()  [unwired: 2 in, 2 out]
          }
        }
        n189 = Get Date/Time String(want seconds? (F)=TRUE) -> (date string=w338:string, time string=w337:string)  [unwired: 2 in]
        n190 = property on="Temperature Readings" class="Clust (strict)"() -> ("Value"=w356:T5)  [unwired: 2 in, 2 out]
        n191 = Bundle By Name(cluster=w356, "HotChamber"=w344, "ColdChamber"=w345, "Date"=w338, "Time"=w337) -> (w355:T5)
        n192 = To Variant(anything=w355) -> (Variant=w354:variant)
        n193 = Bundle("Enum"=StateDef."WriteData", "", "Variant"=w354) -> (w353:cluster{"Enum":T6, string, "Variant":variant})  [unwired: 1 in]
        n194 = Enqueue Element(queue=w342, element=w353, error in (no error)=w341) -> (queue out=w339:refnum<queue>, error out=w350:errorcluster)  [unwired: 1 in, 1 out]
        n195 = property on="UpdateGraph" class="Bool (strict)"(error in=w350, "Value"=TRUE ("UpdateGraph")) -> (error out=w349:errorcluster)  [unwired: 1 in, 1 out]
        n196 = Get Date/Time In Seconds() -> (seconds since 1Jan1904=w351:timestamp)
        n197 = To Unsigned Long Integer(number=w351) -> (unsigned 32bit integer=w352:u32)
        n198 = property on="StartTime" class="DigNum (strict)"(error in=w349, "Value"=w352) -> (error out=w340:errorcluster)  [unwired: 1 in, 1 out]
      }
      frame "AppendFileHeaders" {
        w416 = "\r\n"
        # "Header Section has the following format:\n\nTemperature Readings - File creation date\nSPN #\nData File Path & Name\nTest Name\nCustomer\nOperator\nComments (Operator can add some test parameters here)"
        # "AppendFileHeaders - Message which is queued after the data file is created, this will place all of the header information into the data file before any data is added into the file."
        n199 = property on="Test Information" class="Clust (strict)"() -> ("Value"=w436:T3)  [unwired: 2 in, 2 out]
        n200 = property on="Simulated Data" class="Bool (strict)"() -> ("Value"=w397:bool)  [unwired: 2 in, 2 out]
        n201 = Unbundle By Name(w436) -> ("SPN"=w432:string, "Test Name"=w426:string, "Customer"=w423:string, "Operator"=w421:string, "Comments"=w417:string)
        n202 = case shown="False" w397 {
          tunnel: ["\r\n" w442] -> w395
          frame False {
          }
          frame True {
            n203 = Concatenate Strings(",BasketPosition,", "\r\n") -> (w442:string)
          }
        }
        n204 = Get Date/Time String(want seconds? (F)=TRUE) -> (date string=w404:string, time string=w403:string)  [unwired: 2 in]
        n205 = property on="DataFilePath" class="Path"() -> ("Value"=w437:path)  [unwired: 2 in, 2 out]
        n206 = call <vilib>:"Space Constant.vi"() -> ("String"=w405:string)
        n207 = Path To String(path=w437) -> (string=w429:string)
        n208 = Concatenate Strings("Temperature readings -", w404, w405, w403, "\r\n") -> (w415:string)
        n209 = Concatenate Strings("SPN: ", w432, "\r\n") -> (w414:string)
        n210 = Concatenate Strings("Data File: ", w429, "\r\n") -> (w413:string)
        n211 = Concatenate Strings("Test Name: ", w426, "\r\n") -> (w412:string)
        n212 = Concatenate Strings("Customer:", w423, "\r\n") -> (w411:string)
        n213 = Concatenate Strings("Operator: ", w421, "\r\n") -> (w410:string)
        n214 = Concatenate Strings("Comments: ", w416, w417, w416, w416) -> (w409:string)
        n215 = Concatenate Strings("\r\n", "Date,", "Time,", "Temperature,", w395) -> (w396:string)
        n216 = Concatenate Strings(w415, w414, w413, w412, w411, w410, w409, w396) -> (w408:string)
        n217 = property on="refnum out" class="Ref (strict)"() -> ("Value"=w402:refnum<file>)  [unwired: 2 in, 2 out]
        n218 = Write to Text File(file (use dialog)=w402, text=w408, error in=w407) -> (error out=w439:errorcluster)  [unwired: 1 in, 2 out]
      }
      frame "WriteData" {
        w449 = ","
        # "If the system is in debugging mode (simulated data = true) then the basket state will be written to the data file, otherwise only write the message data."
        # "Message data for the WriteData message is a string cluster with the following structure:\n1. Hot Chamber Temperature\n2. Cold Chamber Temperature\n3. Date\n4. Time\nData is formatted for a csv intput and written to the data file."
        n219 = property on="Simulated Data" class="Bool (strict)"() -> ("Value"=w451:bool)  [unwired: 2 in, 2 out]
        n220 = case shown="True" w451 {
          tunnel: ["\r\n" w473] -> w450
          frame False {
          }
          frame True {
            n221 = property on="Basket Control" class="RadioBtnsControl (strict)"() -> ("Value"=w474:enum32{"Basket Up", "Basket Down"})  [unwired: 2 in, 2 out]
            n222 = Format Into String(w474) -> (resulting string=w471:string)  [unwired: 3 in, 1 out]
            n223 = Concatenate Strings(",", w471, "\r\n") -> (w473:string)
          }
        }
        n224 = Variant To Data(type=cluster{string, string, string, string} {"", "", "", ""}, Variant=w462) -> (data=w461:cluster{string, string, string, string})  [unwired: 1 in, 1 out]
        n225 = Unbundle(w461) -> (w447:string, w446:string, w456:string, w457:string)
        n226 = property on="refnum out" class="Ref (strict)"(error in=w464) -> (error out=w463:errorcluster, "Value"=w465:refnum<file>)  [unwired: 1 in, 1 out]
        n227 = property on="Basket Control" class="RadioBtnsControl (strict)"() -> ("Value"=w448:enum32{"Basket Up", "Basket Down"})  [unwired: 2 in, 2 out]
        n228 = Set File Position(refnum=w465, from (0:start)=enum16{"start", "end", "current"}."end", error in=w463) -> (refnum out=w454:refnum<file>, error out=w455:errorcluster)  [unwired: 1 in]
        n229 = case shown="\"Basket Up\", Default" w448 {
          tunnel: w447 -> [w467 _]
          tunnel: w446 -> [_ w468]
          tunnel: [w467 w468] -> w445
          frame "Basket Up", Default {
          }
          frame "Basket Down" {
          }
        }
        n230 = Concatenate Strings(w457, w449, w456, w449, w445, w449, w450) -> (w452:string)
        n231 = Write to Text File(file (use dialog)=w454, text=w452, error in=w455) -> (error out=w453:errorcluster)  [unwired: 1 in, 2 out]
      }
      frame "CycleBasket" {
        # "Reset the dwell counter and increment the current cyle when the dwell timer ticks."
        # "CycleBasket Message - checks if a true constant is in the message data. If so, this means this message was queued due to the user clicking on the basket control rather than being queued by the software. If the message was queued programatically, then it changes the state of the basket control. If the software is in simulated data mode, then it manually changes the state of the basket control and writes the updated state to an indicator that can be used for debugging. Otherwise it calls the ElevatorControl.VI feeding the appropiate boolean constant depending on the state the basket is coming from."
        n232 = Variant To Data(error in=w479, type=FALSE, Variant=w485) -> (data=w483:bool, error out=w482:errorcluster)
        n233 = case shown="False" w483 {
          tunnel: w482 -> [w500 w508]
          tunnel: [w498 w508] -> w481
          frame False {
            n234 = property on="Basket Control" class="RadioBtnsControl (strict)"(error in=w500) -> (error out=w499:errorcluster, "Value"=w501:enum32{"Basket Up", "Basket Down"})  [unwired: 1 in, 1 out]
            n235 = case shown="\"Basket Up\", Default" w501 {
              tunnel: w499 -> [w503 w506]
              tunnel: [w502 w505] -> w498
              frame "Basket Up", Default {
                n236 = property on="Basket Control" class="RadioBtnsControl (strict)"(error in=w503, "Value"=enum32{"Basket Up", "Basket Down"}."Basket Down" ("Basket Control")) -> (error out=w502:errorcluster)  [unwired: 1 in, 1 out]
              }
              frame "Basket Down" {
                n237 = property on="Basket Control" class="RadioBtnsControl (strict)"(error in=w506, "Value"=enum32{"Basket Up", "Basket Down"}."Basket Up" ("Basket Control")) -> (error out=w505:errorcluster)  [unwired: 1 in, 1 out]
              }
            }
          }
          frame True {
          }
        }
        n238 = property on="Cycling" class="Bool (strict)"(error in=w479) -> (error out=w478:errorcluster, "Value"=w480:bool)  [unwired: 1 in, 1 out]
        n239 = case shown="False" w480 {
          tunnel: w478 -> [w489 w495]
          tunnel: [w489 w490] -> w477
          frame False {
          }
          frame True {
            n240 = Get Date/Time In Seconds() -> (seconds since 1Jan1904=w497:timestamp)
            n241 = To Unsigned Long Integer(number=w497) -> (unsigned 32bit integer=w496:u32)
            n242 = property on="CycleStartTime" class="DigNum (strict)"(error in=w495, "Value"=w496) -> (error out=w492:errorcluster)  [unwired: 1 in, 1 out]
            n243 = property on="CurrentCycle" class="DigNum (strict)"(error in=w492) -> (error out=w491:errorcluster, "Value"=w493:u32)  [unwired: 1 in, 1 out]
            n244 = Increment(x=w493) -> (x+1=w494:u32)
            n245 = property on="CurrentCycle" class="DigNum (strict)"(error in=w491, "Value"=w494) -> (error out=w490:errorcluster)  [unwired: 1 in, 1 out]
          }
        }
        n246 = property on="Simulated Data" class="Bool (strict)"() -> ("Value"=w487:bool)  [unwired: 2 in, 2 out]
        n247 = case shown="False" w487 {
          tunnel: w481 -> [w511 w520]
          tunnel: [w509 w519] -> w475
          frame False {
            n248 = property on="Basket Control" class="RadioBtnsControl (strict)"(error in=w511) -> (error out=w510:errorcluster, "Value"=w512:enum32{"Basket Up", "Basket Down"})  [unwired: 1 in, 1 out]
            n249 = case shown="\"Basket Down\"" w512 {
              tunnel: w510 -> [w515 w518]
              tunnel: [w514 w517] -> w509
              frame "Basket Up", Default {
                n250 = call "ElevatorControl.vi"("error in (no error)"=w515, "Current State IN"=TRUE) -> ("error out"=w514:errorcluster)  [unwired: 7 in, 2 out]
              }
              frame "Basket Down" {
                n251 = call "ElevatorControl.vi"("error in (no error)"=w518, "Current State IN"=FALSE) -> ("error out"=w517:errorcluster)  [unwired: 7 in, 2 out]
              }
            }
          }
          frame True {
            n252 = property on="Basket Control" class="RadioBtnsControl (strict)"(error in=w520) -> (error out=w519:errorcluster, "Value"=→"Basket State":enum32{"Basket Up", "Basket Down"})  [unwired: 1 in, 1 out]
          }
        }
        n253 = Merge Errors(w475, w477) -> (w476:errorcluster)
      }
      frame "ReadInstruments" {
      }
      frame "StopRecording" {
        # "StopRecording - Message which stops the data logging. Updates the states and values of the buttons. If a file was created, then it closes the file."
        n254 = property on="StartRecording" class="Bool"(error in=w531, "DisabledEnum"=T8."Enabled" ("Disabled")) -> (error out=w530:errorcluster)  [unwired: 1 in, 1 out]
        n255 = property on="Stop Recording" class="Bool (strict)"(error in=w530, "DisabledEnum"=T8."Disabled and Grayed Out" ("Disabled")) -> (error out=w529:errorcluster)  [unwired: 1 in, 1 out]
        n256 = property on="Data Recording" class="Bool (strict)"(error in=w529, "Value"=FALSE) -> (error out=w528:errorcluster)  [unwired: 1 in, 1 out]
        n257 = property on="FileCreated" class="Bool (strict)"(error in=w528) -> (error out=w526:errorcluster, "Value"=w527:bool)  [unwired: 1 in, 1 out]
        n258 = case shown="True" w527 {
          tunnel: w526 -> [w537 w542]
          tunnel: [w537 w539] -> w525
          frame False {
          }
          frame True {
            n259 = property on="refnum out" class="Ref (strict)"() -> ("Value"=w541:refnum<file>)  [unwired: 2 in, 2 out]
            n260 = Close File(refnum=w541, error in=w542) -> (error out=w540:errorcluster)  [unwired: 1 out]
            n261 = property on="FileCreated" class="Bool (strict)"(error in=w540, "Value"=FALSE ("FileCreated")) -> (error out=w539:errorcluster)  [unwired: 1 in, 1 out]
          }
        }
      }
      frame "StopCycling" {
        # "StopCycling - Message which stops the cycling of the chamber. Updates the states and values of the cycling buttons."
        n262 = property on="StartCycling" class="Bool (strict)"(error in=w551, "DisabledEnum"=T8."Enabled" ("Disabled")) -> (error out=w550:errorcluster)  [unwired: 1 in, 1 out]
        n263 = property on="StopCycling" class="Bool (strict)"(error in=w550, "DisabledEnum"=T8."Disabled and Grayed Out" ("Disabled")) -> (error out=w545:errorcluster)  [unwired: 1 in, 1 out]
        n264 = property on="StartCycling" class="Bool (strict)"(error in=w545, "Value"=FALSE ("StartCycling")) -> (error out=w544:errorcluster)  [unwired: 1 in, 1 out]
        n265 = property on="Cycling" class="Bool (strict)"(error in=w544, "Value"=FALSE ("Cycling")) -> (error out=w549:errorcluster)  [unwired: 1 in, 1 out]
      }
      frame "TestInformation" {
        # "TestInformation - Message which calls the test information VI. This gives the tech the ability to add the test information paramters. Updates the main panel's data field."
        n266 = call "Input Personal Detail.vi"("Error In"=w558) -> ("Error Out"=w555:errorcluster, "Test Info"=→"Test Information":T12, "Simulated Data?"=→"Simulated Data":bool)  [unwired: 5 in, 1 out]
      }
    }
  }
  n267 = Enqueue Element(queue=w4, element=cluster{"Enum":T6, string, variant} {"Enum"=enum."Initialize", "I have initialzed!", variant}, error in (no error)=w6) -> (queue out=w7:refnum<queue>, error out=w8:errorcluster)  [unwired: 1 in, 1 out]
  n268 = Enqueue Element(queue=w7, element=cluster{"Enum":T6, string, variant} {"Enum"=enum."TestInformation", "", variant}, error in (no error)=w8) -> (queue out=w17:refnum<queue>, error out=w18:errorcluster)  [unwired: 1 in, 1 out]
  n269 = while {
    shift-right: [w562] -> w15
    shift-left: w18 -> [w563]
    tunnel: w17 -> [w564]
    tunnel: [w560] -> _
    stop <- w561 stop-if-true
    # "Event Handler - Enqueue Messages and Data based on UI Inputs"
    n270 = event shown="[10] \"ChamberDwells.min_HotDwell\": Value Change" {
      selector: _ -> [_ _ _ _ _ _ _ _ _ _ _ _ _ _]
      dyn-events: _ -> [_ _ _ _ _ _ _ _ _ _ _ _ _ _]
      timeout: 15 -> [_ _ _ _ _ _ _ _ _ _ _ _ _ _]
      tunnel: w564 -> [_ w569 w573 w607 w611 w621 w630 w658 w673 _ _ _ _ _]
      tunnel: w563 -> [w567 w568 w572 w606 w610 w620 w629 w657 w672 _ w676 w692 w718 w742]
      tunnel: [w567 w568 w570 w605 w609 w618 w628 w655 w670 _ w675 w688 w714 w740] -> w562
      tunnel: [FALSE _ _ _ _ _ TRUE _ _ _ _ _ _ _] -> w561
      tunnel: [_ w569 w571 w603 w608 w619 w627 w656 w671 _ _ _ _ _] -> w560
      event Timeout {
        n271 = event-data() -> ()  [unwired: 1 in, 3 out]
      }
      event "Tab Control": Value Change {
        n272 = event-data() -> ()  [unwired: 1 in, 6 out]
      }
      event "StartRecording": Value Change {
        # "Event to start data recording. Sends a message to the Process Queued Messages loop to start data recording. Includes the recording duration and recording interval as the message data."
        n273 = event-data() -> ()  [unwired: 1 in, 6 out]
        n274 = case shown="True" "StartRecording" {
          tunnel: w573 -> [w576 w584]
          tunnel: w572 -> [w575 w583]
          tunnel: [w576 w581] -> w571
          tunnel: [w575 w580] -> w570
          frame False {
          }
          frame True {
            n275 = Unbundle By Name("Recording Duration") -> ("hours_Duration"=w602:u16, "min_Duration"=w601:u16, "sec_Duration"=w599:i16)
            n276 = Unbundle By Name("Recording Interval") -> ("hours_Interval"=w596:i16, "min_Duration"=w595:i16, "sec_Duration"=w590:i16)
            n277 = Multiply(x=w602, y=3600) -> (x*y=w597:i32)
            n278 = Multiply(x=w601, y=60) -> (x*y=w598:i32)
            n279 = Multiply(x=w596, y=3600) -> (x*y=w592:i32)
            n280 = Multiply(x=w595, y=60) -> (x*y=w591:i32)
            n281 = Compound Arithmetic op=ADD(w597, w598, w599) -> (w589:i32)
            n282 = Compound Arithmetic op=ADD(w592, w591, w590) -> (w588:i32)
            n283 = Build Array(w589, w588) -> (w587:i32[])
            n284 = Bundle("Enum"=StateDef."StartRecording", "", w587) -> (w582:cluster{"Enum":T6, string, i32[]})  [unwired: 1 in]
            n285 = property on="Recording Params" class="Arr (strict)"("Value"=w587) -> ()  [unwired: 2 in, 2 out]
            n286 = Enqueue Element(queue=w584, element=w582, error in (no error)=w583) -> (queue out=w581:refnum<queue>, error out=w580:errorcluster)  [unwired: 1 in, 1 out]
          }
        }
      }
      event "Stop Recording": Value Change {
        # "Event to stop data recording. Sends a message to the Process Queued Messages loop to stop recording data. Eventually can determine if the recording has finished and if not warn the user. Additionally this state happens when duration = recording duration."
        n287 = event-data() -> ()  [unwired: 1 in, 6 out]
        n288 = Enqueue Element(queue=w607, element=cluster{"Enum":T6, string, variant} {"Enum"=enum."StopRecording", "", variant}, error in (no error)=w606) -> (queue out=w603:refnum<queue>, error out=w605:errorcluster)  [unwired: 1 in, 1 out]
      }
      event "StopCycling": Value Change {
        # "Event to stop basket cycling. Sends a message to the Process Queued Messages loop to stop the cycling process. Additionally this state happens when cycles = number of cycles."
        n289 = event-data() -> ()  [unwired: 1 in, 6 out]
        n290 = Enqueue Element(queue=w611, element=cluster{"Enum":T6, string, variant} {"Enum"=enum."StopCycling", "", variant}, error in (no error)=w610) -> (queue out=w608:refnum<queue>, error out=w609:errorcluster)  [unwired: 1 in, 1 out]
      }
      event "Basket Control": Mouse Up {
        # "Event for when user clicks one of the buttons on the basket control panel. Sends the CycleBasket message to the queue, places a True constant in the message data to let the software know that the user has manually adjusted the basket. This is to prevent the indicator from coming desynced from the basket state as the CycleBasket message comes from a couple of different sources."
        n291 = event-data() -> ()  [unwired: 1 in, 8 out]
        n292 = To Variant(anything=TRUE) -> (Variant=w614:variant)
        n293 = Bundle("Enum"=StateDef."CycleBasket", "", "Variant"=w614) -> (w613:cluster{"Enum":T6, string, "Variant":variant})  [unwired: 1 in]
        n294 = Enqueue Element(queue=w621, element=w613, error in (no error)=w620) -> (queue out=w619:refnum<queue>, error out=w618:errorcluster)  [unwired: 1 in, 1 out]
      }
      event Panel Close; "Close Program": Value Change {
        n295 = event-data() -> ()  [unwired: 1 in, 3 out]
        n296 = case shown="True" "Close Program" {
          tunnel: [w633 "Terminate: Close Button Pressed"] -> w626
          frame False {
            n297 = property on="Termination Message" class="Str"() -> ("Value"=w633:string)  [unwired: 2 in, 2 out]
          }
          frame True {
          }
        }
        n298 = Bundle("Enum"=StateDef."Terminate", "Value"=w626, variant) -> (w625:cluster{"Enum":T6, "Value":string, variant})  [unwired: 1 in]
        n299 = Enqueue Element(queue=w630, element=w625, error in (no error)=w629) -> (queue out=w627:refnum<queue>, error out=w628:errorcluster)  [unwired: 1 in, 1 out]
        "Close Data Loop" <- TRUE
      }
      event "StartCycling": Value Change {
        w645 = u32 60
        w646 = u32 3600
        # "Event to start temperature cycling. Sends the StartCycling message to the queue. Includes the dwells in the high and low chambers as well as the number of cycles in the message data."
        n300 = event-data() -> ()  [unwired: 1 in, 1 out]
        n301 = Unbundle By Name("ChamberDwells") -> ("hours_HotDwell"=w652:u32, "min_HotDwell"=w648:u32, "sec_HotDwell"=w642:u32, "sec_ColdDwell"=w641:u32, "min_ColdDwell"=w647:u32, "hours_ColdDwell"=w651:u32)
        n302 = Multiply(x=w652, y=w646) -> (x*y=w662:u32)
        n303 = Multiply(x=w648, y=w645) -> (x*y=w650:u32)
        n304 = Multiply(x=w645, y=w647) -> (x*y=w649:u32)
        n305 = Multiply(x=w651, y=w646) -> (x*y=w661:u32)
        n306 = To Unsigned Long Integer(number=w662) -> (unsigned 32bit integer=w644:u32)
        n307 = To Unsigned Long Integer(number=w650) -> (unsigned 32bit integer=w643:u32)
        n308 = To Unsigned Long Integer(number=w649) -> (unsigned 32bit integer=w640:u32)
        n309 = To Unsigned Long Integer(number=w661) -> (unsigned 32bit integer=w639:u32)
        n310 = Compound Arithmetic op=ADD(w641, w640, w639) -> (w637:u32)
        n311 = Compound Arithmetic op=ADD(w644, w643, w642) -> (w638:u32)
        n312 = property on="Number of Cycles" class="DigNum (strict)"() -> ("Value"=w635:u32)  [unwired: 2 in, 2 out]
        n313 = Build Array(w638, w637, w635) -> (w636:u32[])
        n314 = Bundle("Enum"=StateDef."StartCycling", "", w636) -> (w654:cluster{"Enum":T6, string, u32[]})  [unwired: 1 in]
        n315 = Enqueue Element(queue=w658, element=w654, error in (no error)=w657) -> (queue out=w656:refnum<queue>, error out=w655:errorcluster)  [unwired: 1 in, 1 out]
      }
      event "ProgramTemp": Value Change {
        n316 = event-data() -> ()  [unwired: 1 in, 6 out]
        n317 = property on="HotSetPoint" class="DigNum (strict)"() -> ("Value"=w669:i32)  [unwired: 2 in, 2 out]
        n318 = property on="ColdSetPoint" class="DigNum (strict)"() -> ("Value"=w668:i32)  [unwired: 2 in, 2 out]
        n319 = Bundle("Value"=w669, "Value"=w668) -> (w667:cluster{"Value":i32, "Value":i32})  [unwired: 1 in]
        n320 = To Variant(anything=w667) -> (Variant=w664:variant)
        n321 = Bundle("Enum"=StateDef."ProgramTemperatures", "", "Variant"=w664) -> (w663:cluster{"Enum":T6, string, "Variant":variant})  [unwired: 1 in]
        n322 = Enqueue Element(queue=w673, element=w663, error in (no error)=w672) -> (queue out=w671:refnum<queue>, error out=w670:errorcluster)  [unwired: 1 in, 1 out]
      }
      event Panel Close? {
        n323 = event-data() -> ()  [unwired: 1 in, 4 out]
        n324 = property on="Termination Message" class="Str"("Value"="Program terminated by pressing \"Close Program\" button in main VI!") -> ()  [unwired: 2 in, 2 out]
        n325 = event-data() -> ()  [unwired: 2 in, 1 out]
      }
      event "ChamberDwells.min_HotDwell": Value Change {
        # "Event to handle chamber dwell control. If the user uses the up-arrow control when the value is set to 59 it will reset the control to 0 and increment the hours control."
        n326 = event-data() -> ("OldVal"=w678:u32)  [unwired: 1 in, 5 out]
        n327 = Equal?(x=w678, y=u32 59) -> (x = y?=w677:bool)
        n328 = case shown="True" w677 {
          tunnel: w676 -> [w680 w684]
          tunnel: [w680 w681] -> w675
          frame False {
          }
          frame True {
            n329 = property on="min_HotDwell" class="DigNum (strict)"(error in=w684, "Value"=u32 0) -> (error out=w683:errorcluster)  [unwired: 1 in, 1 out]
            n330 = property on="hours_HotDwell" class="DigNum (strict)"(error in=w683) -> (error out=w682:errorcluster, "Value"=w686:u32)  [unwired: 1 in, 1 out]
            n331 = Increment(x=w686) -> (x+1=w685:u32)
            n332 = property on="hours_HotDwell" class="DigNum (strict)"(error in=w682, "Value"=w685) -> (error out=w681:errorcluster)  [unwired: 1 in, 1 out]
          }
        }
      }
      event "ChamberDwells.sec_ColdDwell": Value Change {
        # "Event to handle chamber dwell control. If the user uses the up-arrow control when the value is set to 59 it will reset the control to 0 and increment the minutes control, if this increments the minutes control passed 59 then reset the minutes and increment the hours."
        n333 = event-data() -> ("OldVal"=w691:u32)  [unwired: 1 in]
        n334 = Equal?(x=w691, y=u32 59) -> (x = y?=w689:bool)
        n335 = case shown="True" w689 {
          tunnel: w692 -> [w693 w704]
          tunnel: [w693 w694] -> w688
          frame False {
          }
          frame True {
            n336 = property on="sec_ColdDwell" class="DigNum (strict)"(error in=w704, "Value"=u32 0) -> (error out=w703:errorcluster)  [unwired: 1 in, 1 out]
            n337 = property on="min_ColdDwell" class="DigNum (strict)"(error in=w703) -> (error out=w702:errorcluster, "Value"=w700:u32)  [unwired: 1 in, 1 out]
            n338 = Increment(x=w700) -> (x+1=w701:u32)
            n339 = property on="min_ColdDwell" class="DigNum (strict)"(error in=w702, "Value"=w701) -> (error out=w699:errorcluster)  [unwired: 1 in, 1 out]
            n340 = property on="min_ColdDwell" class="DigNum (strict)"(error in=w699) -> (error out=w695:errorcluster, "Value"=w698:u32)  [unwired: 1 in, 1 out]
            n341 = Equal?(x=w698, y=u32 60) -> (x = y?=w696:bool)
            n342 = case shown="True" w696 {
              tunnel: w695 -> [w706 w712]
              tunnel: [w706 w709] -> w694
              frame False {
              }
              frame True {
                n343 = property on="min_ColdDwell" class="DigNum (strict)"(error in=w712, "Value"=u32 0) -> (error out=w711:errorcluster)  [unwired: 1 in, 1 out]
                n344 = property on="hours_ColdDwell" class="DigNum (strict)"(error in=w711) -> (error out=w710:errorcluster, "Value"=w708:u32)  [unwired: 1 in, 1 out]
                n345 = Increment(x=w708) -> (x+1=w707:u32)
                n346 = property on="hours_ColdDwell" class="DigNum (strict)"(error in=w710, "Value"=w707) -> (error out=w709:errorcluster)  [unwired: 1 in, 1 out]
              }
            }
          }
        }
      }
      event "ChamberDwells.sec_HotDwell": Value Change {
        # "Event to handle chamber dwell control. If the user uses the up-arrow control when the value is set to 59 it will reset the control to 0 and increment the minutes control."
        n347 = event-data() -> ("OldVal"=w717:u32)  [unwired: 1 in]
        n348 = Equal?(x=w717, y=u32 59) -> (x = y?=w715:bool)
        n349 = case shown="True" w715 {
          tunnel: w718 -> [w719 w725]
          tunnel: [w719 w720] -> w714
          frame False {
          }
          frame True {
            n350 = property on="sec_HotDwell" class="DigNum (strict)"(error in=w725, "Value"=u32 0) -> (error out=w724:errorcluster)  [unwired: 1 in, 1 out]
            n351 = property on="min_HotDwell" class="DigNum (strict)"(error in=w724) -> (error out=w723:errorcluster, "Value"=w731:u32)  [unwired: 1 in, 1 out]
            n352 = Increment(x=w731) -> (x+1=w730:u32)
            n353 = property on="min_HotDwell" class="DigNum (strict)"(error in=w723, "Value"=w730) -> (error out=w722:errorcluster)  [unwired: 1 in, 1 out]
            n354 = property on="min_HotDwell" class="DigNum (strict)"(error in=w722) -> (error out=w721:errorcluster, "Value"=w728:u32)  [unwired: 1 in, 1 out]
            n355 = Equal?(x=w728, y=u32 60) -> (x = y?=w727:bool)
            n356 = case shown="False" w727 {
              tunnel: w721 -> [w732 w736]
              tunnel: [w732 w733] -> w720
              frame False {
              }
              frame True {
                n357 = property on="min_HotDwell" class="DigNum (strict)"(error in=w736, "Value"=u32 0) -> (error out=w735:errorcluster)  [unwired: 1 in, 1 out]
                n358 = property on="hours_HotDwell" class="DigNum (strict)"(error in=w735) -> (error out=w734:errorcluster, "Value"=w738:u32)  [unwired: 1 in, 1 out]
                n359 = Increment(x=w738) -> (x+1=w737:u32)
                n360 = property on="hours_HotDwell" class="DigNum (strict)"(error in=w734, "Value"=w737) -> (error out=w733:errorcluster)  [unwired: 1 in, 1 out]
              }
            }
          }
        }
      }
      event "ChamberDwells.min_ColdDwell": Value Change {
        # "Event to handle chamber dwell control. If the user uses the up-arrow control when the value is set to 59 it will reset the control to 0 and increment the minutes control."
        n361 = event-data() -> ("OldVal"=w744:u32)  [unwired: 1 in, 5 out]
        n362 = Equal?(x=w744, y=u32 59) -> (x = y?=w741:bool)
        n363 = case shown="True" w741 {
          tunnel: w742 -> [w745 w751]
          tunnel: [w745 w746] -> w740
          frame False {
          }
          frame True {
            n364 = property on="min_ColdDwell" class="DigNum (strict)"(error in=w751, "Value"=u32 0) -> (error out=w748:errorcluster)  [unwired: 1 in, 1 out]
            n365 = property on="hours_ColdDwell" class="DigNum (strict)"(error in=w748) -> (error out=w747:errorcluster, "Value"=w750:u32)  [unwired: 1 in, 1 out]
            n366 = Increment(x=w750) -> (x+1=w749:u32)
            n367 = property on="hours_ColdDwell" class="DigNum (strict)"(error in=w747, "Value"=w749) -> (error out=w746:errorcluster)  [unwired: 1 in, 1 out]
          }
        }
      }
    }
  }
  n368 = Merge Errors(w15, w14) -> (w12:errorcluster)
  n369 = property on="Simulated Data" class="Bool (strict)"() -> ("Value"=w11:bool)  [unwired: 2 in, 2 out]
  n370 = Release Queue(queue=w13, error in (no error)=w12) -> (error out=w10:errorcluster)  [unwired: 1 in, 2 out]
  n371 = case shown="True" w11 {
    tunnel: w10 -> [w753 w754]
    tunnel: [w753 w754] -> w9
    frame False {
    }
    frame True {
    }
  }
  "error out" <- w9
